vi "FindNewAxis 8.6.vi"(5 "Angle":sgl, 6 "Y":dbl, 7 "Z":dbl, 8 "X":dbl=1.0, 9 "Axis":cluster{"X":sgl, "Y":sgl, "Z":sgl}) -> (2 "New Axis":cluster{"X":sgl, "Y":sgl, "Z":sgl})   [LabVIEW 2016]
uses:
  <vilib>/Analysis/Matrix/Numeric/Conversions/Array To Matrix - RA2.vi
  <vilib>/Analysis/Matrix/Numeric/Multiply/Multiply - RM,RM.vi
  <vilib>/Analysis/Matrix/NI_Matrix.lvlib
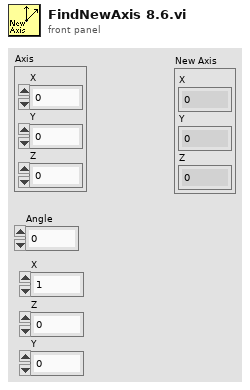
[diagram p1: front panel]
types:
  T1 = typedef "NI_Matrix.lvlib/RealMatrix.ctl" = dbl[][]
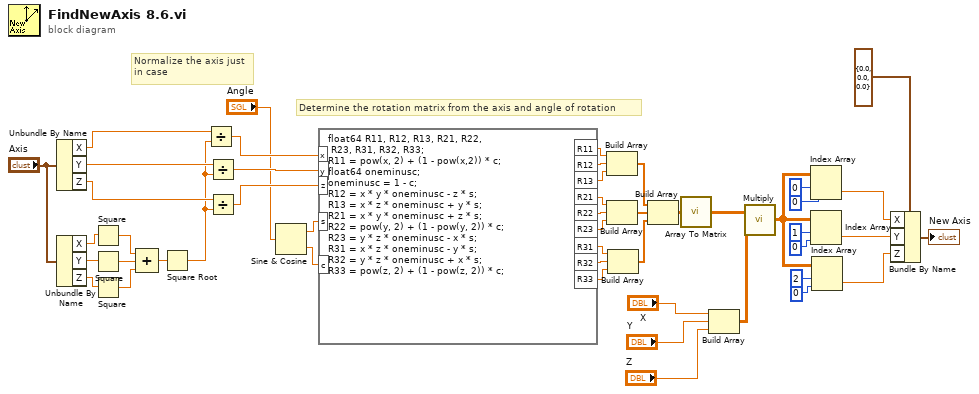
[diagram p0: block diagram]
diagram:
  # "Normalize the axis just\nin case"
  # "Determine the rotation matrix from the axis and angle of rotation"
  n1 = Unbundle By Name("Axis") -> ("X"=w10:sgl, "Y"=w8:sgl, "Z"=w7:sgl)
  n2 = Unbundle By Name("Axis") -> ("X"=w18:sgl, "Y"=w17:sgl, "Z"=w16:sgl)
  n3 = Square(x=w18) -> (x^2=w15:sgl)
  n4 = Square(x=w17) -> (x^2=w14:sgl)
  n5 = Square(x=w16) -> (x^2=w13:sgl)
  n6 = Compound Arithmetic op=ADD(w15, w14, w13) -> (w12:sgl)
  n7 = Square Root(x=w12) -> (sqrt(x)=w6:sgl)
  n8 = Divide(x=w10, y=w6) -> (x/y=w9:sgl)
  n9 = Divide(x=w8, y=w6) -> (x/y=w5:sgl)
  n10 = Divide(x=w7, y=w6) -> (x/y=w4:sgl)
  n11 = Sine & Cosine(0:"Angle") -> (1:w2:sgl, 2:w1:sgl)
  n12 = formula code="float64 R11, R12, R13, R21, R22,\n R23, R31, R32, R33;\nR11 = pow(x, 2) + (1 - pow(x,2)) * c;\nfloat64 oneminusc;\noneminusc = 1 - c;\nR12 = x * y * oneminusc - z * s;\nR13 = x * z * oneminusc + y * s;\nR21 = x * y * oneminusc + z * s;\nR22 = pow(y, 2) + (1 - pow(y, 2)) * c;\nR23 = y * z * oneminusc - x * s;\nR31 = x * z * oneminusc - y * s;\nR32 = y * z * oneminusc + x * s;\nR33 = pow(z, 2) + (1 - pow(z, 2)) * c;"("x"=w9, "y"=w5, "z"=w4, "s"=w2, "c"=w1) -> ("R11"=w36:dbl, "R12"=w37:dbl, "R13"=w38:dbl, "R21"=w39:dbl, "R22"=w40:dbl, "R23"=w41:dbl, "R31"=w42:dbl, "R32"=w43:dbl, "R33"=w44:dbl)
  n13 = Build Array(w36, w37, w38) -> (w46:dbl[])
  n14 = Build Array(w39, w40, w41) -> (w45:dbl[])
  n15 = Build Array(w42, w43, w44) -> (w47:dbl[])
  n16 = Build Array(w46, w45, w47) -> (w48:dbl[][])
  n17 = call-poly <vilib>:"Array To Matrix.vi"("Real 2D Array"=w48) -> ("Real Matrix"=w29:T1)
  n18 = Build Array("X", "Y", "Z") -> (w33:T1)
  n19 = call-poly <vilib>:"Multiply.vi"("Real Matrix B"=w33, "Real Matrix A"=w29) -> ("A * B"=w24:T1)
  n20 = Index Array(array=w24, index (row)=0, index (col)=0) -> (element=w22:dbl)
  n21 = Index Array(array=w24, index (row)=1, index (col)=0) -> (element=w21:dbl)
  n22 = Index Array(array=w24, index (row)=2, index (col)=0) -> (element=w20:dbl)
  n23 = Bundle By Name(cluster=cluster{"X":sgl, "Y":sgl, "Z":sgl} {"X"=0.0, "Y"=0.0, "Z"=0.0} ("Axis"), "X"=w22, "Y"=w21, "Z"=w20) -> (→"New Axis":cluster{"X":sgl, "Y":sgl, "Z":sgl})
